vi "Write Grant Type.vi"(8 "error in (no error)":errorcluster, 10 "Grant Type (authorization_code)":T1="authorization_code", 11 "Oauth2 in":refnum<class "Oauth2.lvclass">) -> (0 "error out":errorcluster, 3 "Oauth2 out":refnum<class "Oauth2.lvclass">)   [LabVIEW 2017, in "Oauth2.lvclass"]
doc: "The default grant_type is authorization_code. <B>grant_type</B> is a REQUIRED parameter that is associated with a Grant Flow.\n\nIf the grant_type is unwired, the current Oauth2 <B>Grant Flow</B> value (Authorization Code) will be used to set the grant_type."
uses:
  Oauth2.lvclass
  OAuth2 Grant Type -- ring.ctl
  Oauth2.lvclass/Oauth2.ctl
  OAuth2 Flow -- enum.ctl
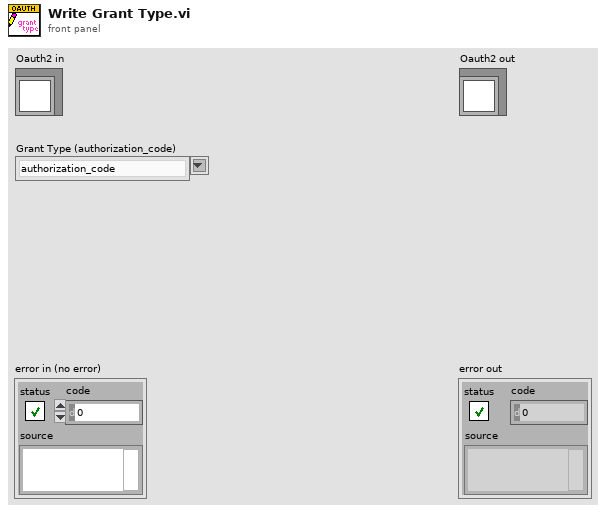
[diagram p1: front panel]
types:
  T1 = typedef "Oauth2.lvclass/OAuth2 Grant Type -- ring.ctl" = string
  T2 = typedef "Oauth2.lvclass/OAuth2 Flow -- enum.ctl" = enum16{"Authorization Code", "Authorization Code (PKCE)", "Implicit", "Resource Owner Credentials", "Client Credentials", "Refresh Token", "Device Code"}
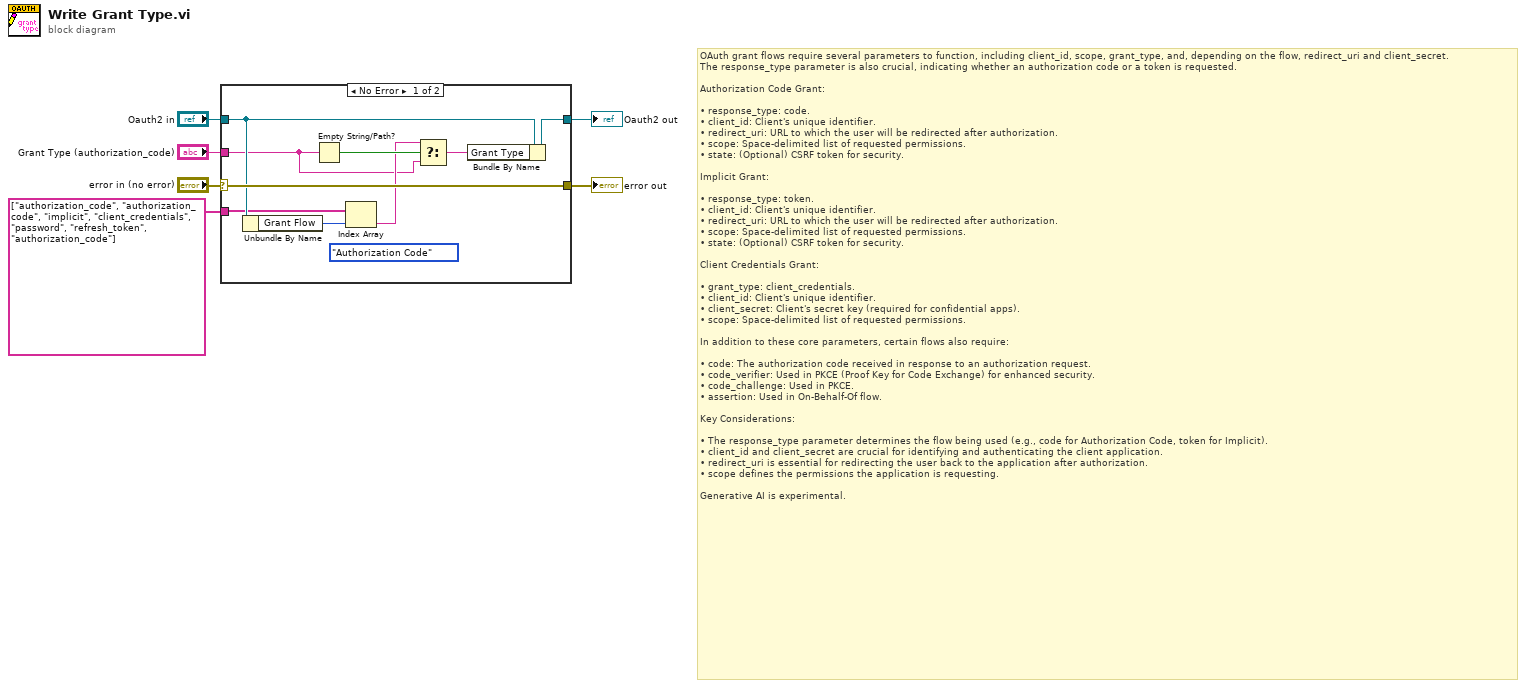
[diagram p0: block diagram]
diagram:
  # "OAuth grant flows require several parameters to function, including client_id, scope, grant_type, and, depending on the flow, redirect_uri and client_secret. \nThe response_type parameter is also crucial, indicating whether an authorization code or a token is requested.\n\nAuthorization Code Grant: \n\n• response_type: code. \n• client_id: Client's unique identifier. \n• redirect_uri: URL to which the user will be redirected after authorization. \n• scope: Space-delimited list of requested permissions. \n• state: (Optional) CSRF token for security. \n\nImplicit Grant: \n\n• response_type: token. \n• client_id: Client's unique identifier. \n• redirect_uri: URL to which the user will be redirected after authorization. \n• scope: Space-delimited list of requested permissions. \n• state: (Optional) CSRF token for security. \n\nClient Credentials Grant: \n\n• grant_type: client_credentials. \n• client_id: Client's unique identifier. \n• client_secret: Client's secret key (required for confidential apps). \n• scope: Space-delimited list of requested permissions. \n\nIn addition to these core parameters, certain flows also require: \n\n• code: The authorization code received in response to an authorization request. \n• code_verifier: Used in PKCE (Proof Key for Code Exchange) for enhanced security. \n• code_challenge: Used in PKCE. \n• assertion: Used in On-Behalf-Of flow. \n\nKey Considerations: \n\n• The response_type parameter determines the flow being used (e.g., code for Authorization Code, token for Implicit). \n• client_id and client_secret are crucial for identifying and authenticating the client application. \n• redirect_uri is essential for redirecting the user back to the application after authorization. \n• scope defines the permissions the application is requesting. \n\nGenerative AI is experimental."
  n1 = case shown="No Error" "error in (no error)" {
    selector: "error in (no error)" -> [w15 w16]
    tunnel: [w15 w16] -> w5
    tunnel: [w14 w17] -> w3
    tunnel: "Oauth2 in" -> [w13 w17]
    tunnel: "Grant Type (authorization_code)" -> [w8 _]
    tunnel: T1[] ["authorization_code", "authorization_code", "implicit", "client_credentials", "password", "refresh_token", "authorization_code"] -> [w11 _]
    frame No Error {
      (unwired) OAuth2_Flow_--_enum."Authorization Code" ("Grant Flow")
      n2 = Unbundle By Name(w13) -> ("Grant Flow"=w10:T2)
      n3 = Empty String/Path?(string/path=w8) -> (empty?=w12:bool)
      n4 = Index Array(array=w11, index=w10) -> (element=w9:T1)
      n5 = Select(t=w9, s=w12, f=w8) -> (s? t:f=w7:T1)
      n6 = Bundle By Name(cluster=w13, "Grant Type"=w7) -> (w14:refnum<class "Oauth2.lvclass">)
    }
    frame Error {
    }
  }
  "error out" <- w5
  "Oauth2 out" <- w3
